vi "Read Profile.vi"(7 "Refresh":bool, 9 "FPGA Name":string, 10 "Channel to Read":T2, 11 "myRIO PID":string) -> (2 "Channel List Out":T3[](array[typedef]), 3 "Profile Data Out":T1[](array[typedef]))   [LabVIEW 2021]
uses:
  <vilib>/myRIO/Common/Profile Manager Framework/typedefs/Channel Type Profile.ctl
  <vilib>/myRIO/Common/Instrument Driver Framework/Utilities/typedefs/Channel Types.ctl
  <vilib>/myRIO/Common/Profile Manager Framework/typedefs/Channel Info.ctl
panel:
  out "Channel Type Profile Out":T1
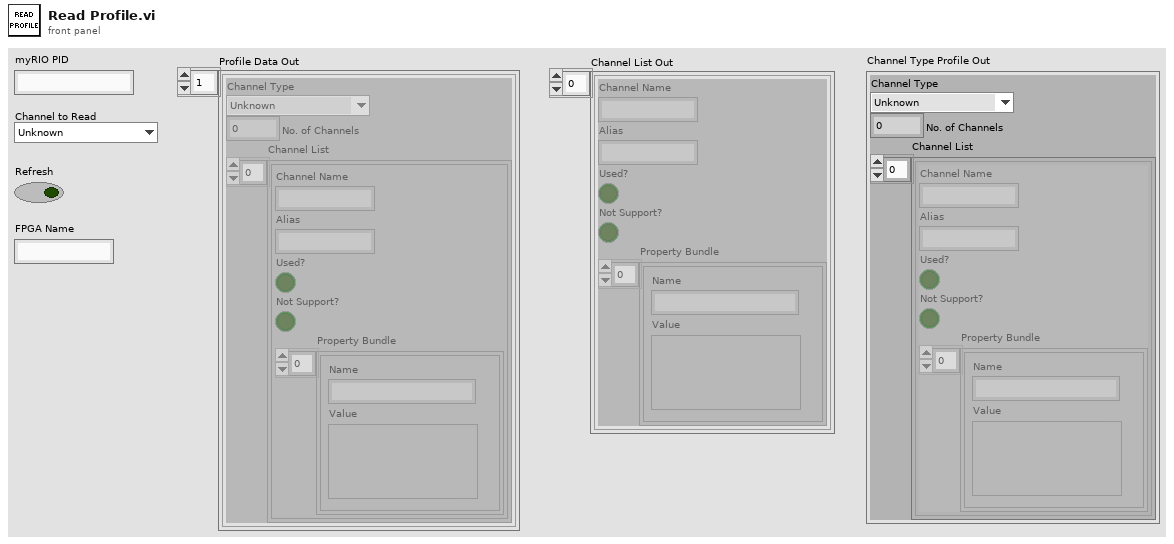
[diagram p1: front panel]
types:
  T1 = typedef "Channel Type Profile.ctl" = cluster{"Channel Type":T2, "No. of Channels":dbl, "Channel List":T3[]}
  T2 = typedef "Channel Types.ctl" = enum32{"Unknown", "AI", "AO", "DIO - DI", "DIO", "DIO - DO", "I2C", "PWM", "Encoder", "SPI", "UART", "Accelerometer", "DIO - LED", "DIO - Button", "AI (N Samples)", "AudioIn (N Samples)", "AO (N Samples)", "AudioOut (N Samples)", "DI (N Samples)", "DO (N Samples)", "AI IRQ", "DI IRQ", "Timer IRQ", "RSL", "Relay", "CAN", "AI (Continuous)", "AO (Continuous)"}
  T3 = typedef "Channel Info.ctl" = cluster{"Channel Name":string, "Alias":string, "Used?":bool, "Not Support?":bool, "Property Bundle":cluster{"Name":string, "Value":variant}[]}
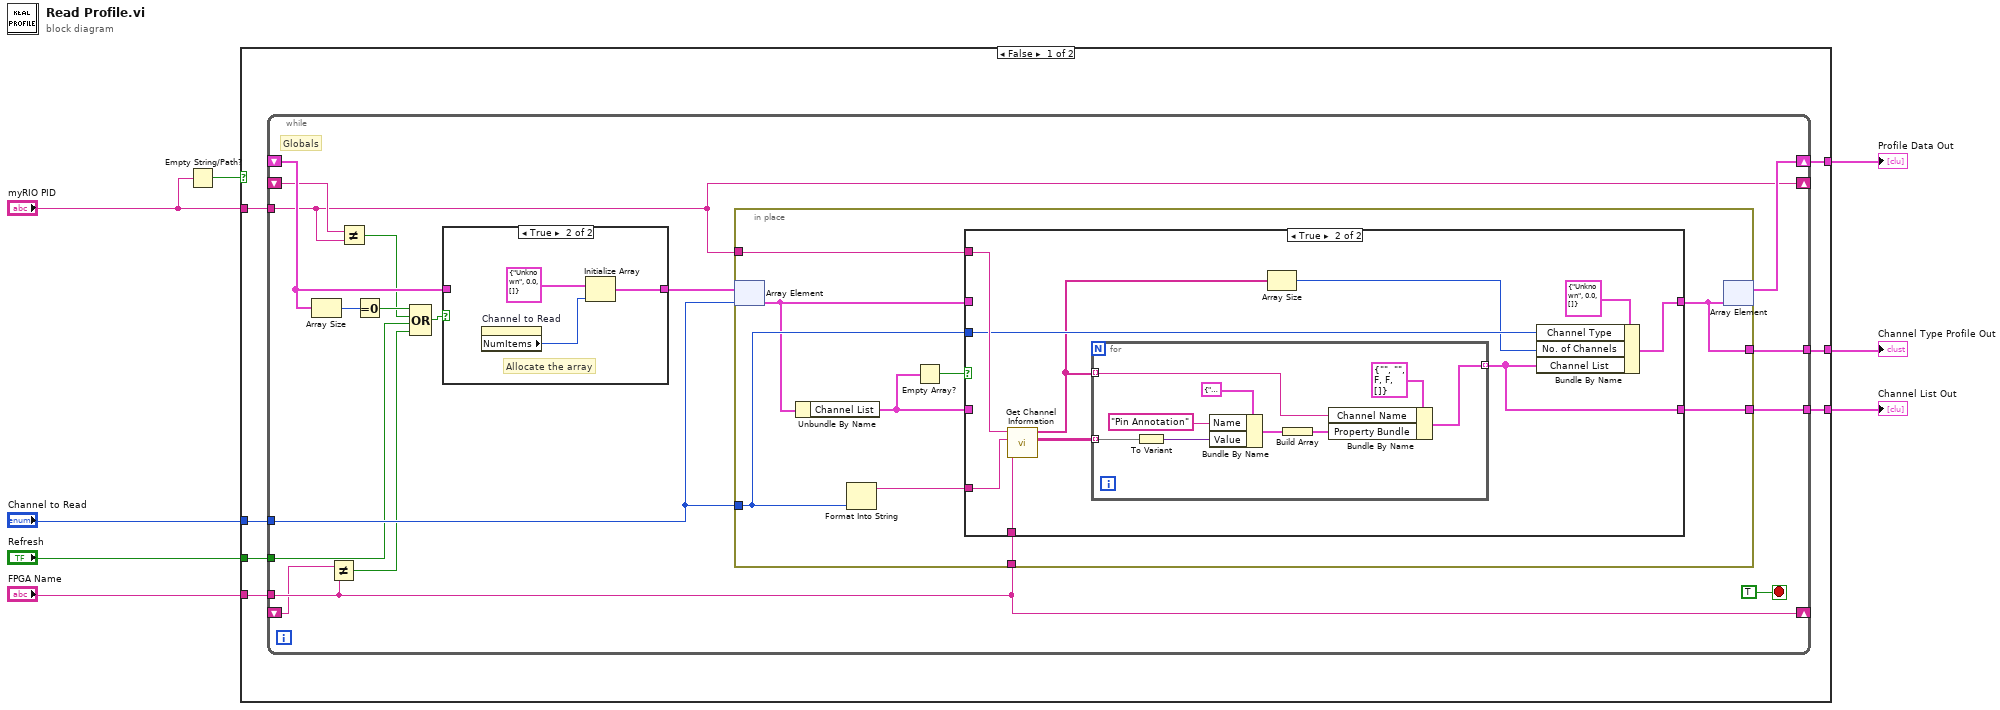
[diagram p0: block diagram]
diagram:
  n1 = Empty String/Path?(string/path="myRIO PID") -> (empty?=w2:bool)
  n2 = case shown="False" w2 {
    tunnel: [w15 _] -> w8
    tunnel: [w14 _] -> w7
    tunnel: "Channel to Read" -> [w13 _]
    tunnel: "Refresh" -> [w12 _]
    tunnel: [w11 _] -> w4
    tunnel: "myRIO PID" -> [w10 _]
    tunnel: "FPGA Name" -> [w9 _]
    frame False {
      n3 = while {
        shift-right: [w23] -> w14
        shift-left: _ -> [w26]
        tunnel: w13 -> [w29]
        tunnel: w10 -> [w20]
        tunnel: [w28] -> w15
        tunnel: w12 -> [w24]
        tunnel: [w22] -> w11
        shift-right: [w20] -> _
        shift-left: _ -> [w21]
        tunnel: w9 -> [w18]
        shift-right: [w18] -> _
        shift-left: _ -> [w17]
        stop <- TRUE stop-if-true
        # "Globals"
        n4 = Array Size(array=w26) -> (size(s)=w31:i32)
        n5 = Not Equal?(x=w17, y=w18) -> (x != y?=w16:bool)
        n6 = Not Equal?(x=w21, y=w20) -> (x != y?=w19:bool)
        n7 = Equal To 0?(x=w31) -> (x = 0?=w30:bool)
        n8 = Compound Arithmetic op=OR(w30, w19, w24, w16) -> (w27:bool)
        n9 = case shown="True" w27 {
          tunnel: [w63 w64] -> w25
          tunnel: w26 -> [w63 _]
          frame False {
          }
          frame True {
            # "Allocate the array"
            n10 = property on="Channel to Read" class="Enum (strict)"() -> ("NumItems"=w65:u32)  [unwired: 2 in, 2 out]
            n11 = Initialize Array(T1 {"Channel Type"=enum."Unknown", "No. of Channels"=0.0, "Channel List"=[]} ("Channel Type Profile Out"), w65) -> (w64:T1[])
          }
        }
        n12 = in-place {
          in-place-border: w20 -> [w40]
          in-place-border: w29 -> [w39]
          in-place-border: [w36] -> w28
          in-place-border: [w35] -> w22
          in-place-border: w18 -> [w33]
          n13 = in-place-array #1(w25, w29) -> (w37:T1)
          n14 = Unbundle By Name(w37) -> ("Channel List"=w34:T3[])
          n15 = Format Into String(w39) -> (resulting string=w41:string)  [unwired: 3 in, 1 out]
          n16 = Empty Array?(array=w34) -> (empty?=w38:bool)
          n17 = case shown="True" w38 {
            tunnel: w41 -> [_ w53]
            tunnel: w40 -> [_ w52]
            tunnel: w39 -> [_ w51]
            tunnel: w37 -> [w43 _]
            tunnel: [w43 w46] -> w36
            tunnel: [w42 w45] -> w35
            tunnel: w34 -> [w42 _]
            tunnel: w33 -> [_ w44]
            frame False {
            }
            frame True {
              n18 = call <vilib>:"Get Channel Information.vi"("FPGA Name"=w44, "Channel Type"=w53, "myRIO PID"=w52) -> ("Pin Info"=w47:string[][], "Channel List"=w48:string[])  [unwired: 7 in]
              n19 = for {
                tunnel: w48 -> [w61] mode=indexing
                tunnel: [w60] -> w45 mode=indexing
                tunnel: w47 -> [w57] mode=indexing
                n20 = To Variant(anything=w57) -> (Variant=w56:variant)
                n21 = Bundle By Name(cluster=cluster{"Name":string, "Value":variant} {"Name"="", "Value"=variant} ("Property"), "Name"="Pin Annotation", "Value"=w56) -> (w55:cluster{"Name":string, "Value":variant})
                n22 = Build Array(w55) -> (w54:cluster{"Name":string, "Value":variant}[])
                n23 = Bundle By Name(cluster=T3 {"Channel Name"="", "Alias"="", "Used?"=FALSE, "Not Support?"=FALSE, "Property Bundle"=[]} ("Channel Info"), "Channel Name"=w61, "Property Bundle"=w54) -> (w60:T3)
              }
              n24 = Array Size(array=w48) -> (size(s)=w50:i32)
              n25 = Bundle By Name(cluster=T1 {"Channel Type"=enum."Unknown", "No. of Channels"=0.0, "Channel List"=[]} ("Channel Type Profile Out"), "Channel Type"=w51, "No. of Channels"=w50, "Channel List"=w45) -> (w46:T1)
            }
          }
          n26 = in-place-array #1(w36) -> (w23:T1[])  [unwired: 1 out]
        }
      }
    }
    frame True {
    }
  }
  "Channel Type Profile Out" <- w8
  "Channel List Out" <- w4
  "Profile Data Out" <- w7
